vi "GenerateValidTagSettings.vi"(6 "Minimum tagging period (pws)":u32, 7 "PulseWidth (ms)":dbl, 9 "Minimum tags per file":u32, 10 "Minimum samples per pulse":dbl) -> (0 "TaggingPeriod (pws)":u32, 3 "Valid Pulse Width (ms)":dbl)   [LabVIEW 2015]
uses:
  <vilib>/Utility/error.llb/DialogType.ctl
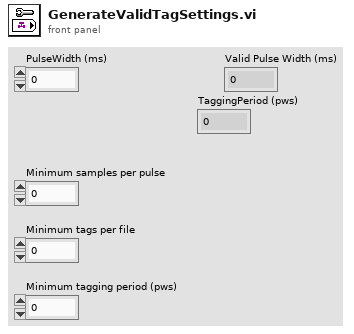
[diagram p1: front panel]
types:
  T1 = typedef "DialogType.ctl" = u16
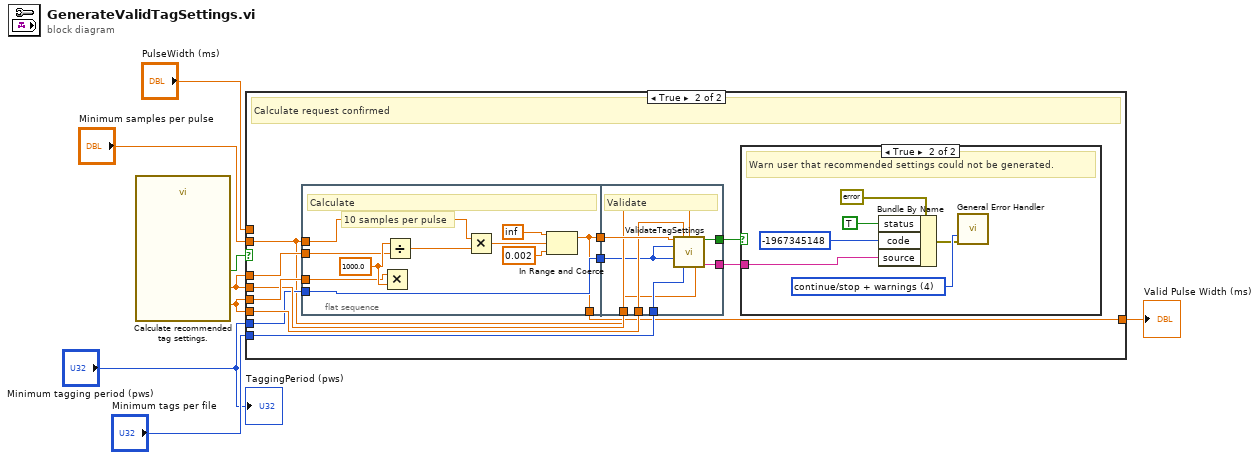
[diagram p0: block diagram]
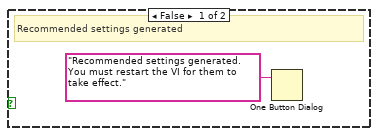
[diagram p3: hidden frame]
diagram:
  n1 = call "Calculate recommended tag settings."() -> ("Minimum file size (s)"=w3:dbl, "Minimum sampling rate (Hz)"=w4:dbl, "Calculate"=w2:bool)  [unwired: 16 in, 1 out]
  n2 = case shown="True" w2 {
    tunnel: w3 -> [_ w21]
    tunnel: w3 -> [_ w18]
    tunnel: w4 -> [_ w17]
    tunnel: w4 -> [_ w15]
    tunnel: "Minimum tagging period (pws)" -> [_ w13]
    tunnel: "Minimum tags per file" -> [_ w12]
    tunnel: "Minimum samples per pulse" -> [_ w10]
    tunnel: [w9 w11] -> w7
    tunnel: "PulseWidth (ms)" -> [w9 _]
    frame False {
    }
    frame True {
      # "Calculate request confirmed"
      n3 = flat-sequence {
        tunnel: w21 -> [w26]
        tunnel: w17 -> [w25]
        tunnel: [w22] -> w20
        tunnel: [w23] -> w19
        tunnel: w10 -> [w24]
        tunnel: w13 -> [w23]
        tunnel: [w22] -> w11
        tunnel: w20 -> [w39]
        tunnel: w19 -> [w34]
        tunnel: w18 -> [w38]
        tunnel: [w37] -> w16
        tunnel: w15 -> [w36]
        tunnel: [w35] -> w14
        tunnel: w12 -> [w33]
        tunnel: w10 -> [w32]
        frame #0 {
          w30 = 1000.0
          # "10 samples per pulse"
          # "Calculate"
          n4 = Multiply(x=w26, y=w30) -> ()  [unwired: 1 out]
          n5 = Divide(x=w30, y=w25) -> (x/y=w31:dbl)
          n6 = Multiply(x=w24, y=w31) -> (x*y=w27:dbl)
          n7 = In Range and Coerce(upper limit=inf, x=w27, lower limit=0.002) -> (coerced(x)=w22:dbl)  [unwired: 1 out]
        }
        frame #1 {
          # "Validate"
          n8 = call "ValidateTagSettings.vi"("PulseWidth (ms)"=w39, "Minimum file size (s)"=w38, "Minimum sample rate (Hz)"=w36, "TaggingPeriod (pws)"=w34, "Minimum tagging period (pws)"=w34, "Minimum tags per file"=w33, "Minimum samples per pulse"=w32) -> ("Valid"=w37:bool, "Info"=w35:string)  [unwired: 7 in]
        }
      }
      n9 = case shown="True" w16 {
        tunnel: w14 -> [_ w41]
        frame False {
          # "Recommended settings generated"
          n10 = One Button Dialog(message="Recommended settings generated. You must restart the VI for them to take effect.") -> ()  [unwired: 1 in, 1 out]
        }
        frame True {
          w46 = T1 4 items=["no dialog", "OK message", "continue or stop message", "OK message + warnings", "continue/stop + warnings"] ("type of dialog (OK msg:1)")
          # "Warn user that recommended settings could not be generated."
          n11 = Bundle By Name(cluster=errorcluster {"status"=FALSE, "code"=0, "source"=""} ("error in (no error)"), "status"=TRUE, "code"=-1967345148, "source"=w41) -> (w45:errorcluster)
          n12 = call <vilib>:"General Error Handler.vi"("type of dialog (OK msg:1)"=w46, "error in (no error)"=w45) -> ()  [unwired: 9 in, 5 out]
        }
      }
    }
  }
  "Valid Pulse Width (ms)" <- w7
  "TaggingPeriod (pws)" <- "Minimum tagging period (pws)"
